vi "BeamLocWrapper.vi"(10 "Beam Location":cluster{"X":dbl, "Y":dbl}, 11 "DLLpath":path) -> ()   [LabVIEW 2014]
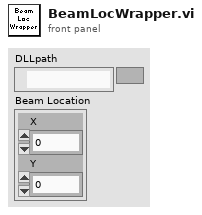
[diagram p1: front panel]
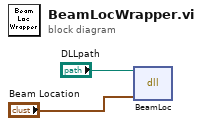
[diagram p0: block diagram]
diagram:
  n1 = dll-call lib="C:/Users/guss2/Desktop/GVI/Git/LVslicer/MachineController/DLL/MachineSimulator.dll" fn="BeamLoc"(path in="DLLpath", "BeamLoc"="Beam Location") -> ()  [unwired: 4 in, 2 out]
